vi "TesteTR4CS.vi"() -> ()   [LabVIEW 2024]
uses:
  <vilib>/DAQmx/read.llb/DAQmx Read (Analog DBL 1Chan 1Samp).vi
  <vilib>/DAQmx/miscellaneous.llb/DAQmx Fill In Error Info.vi
panel:
  out "Waveform Chart 3":dbl(graph)
  out "Waveform Chart 2":dbl(graph)
  out "Waveform Chart":dbl(graph)
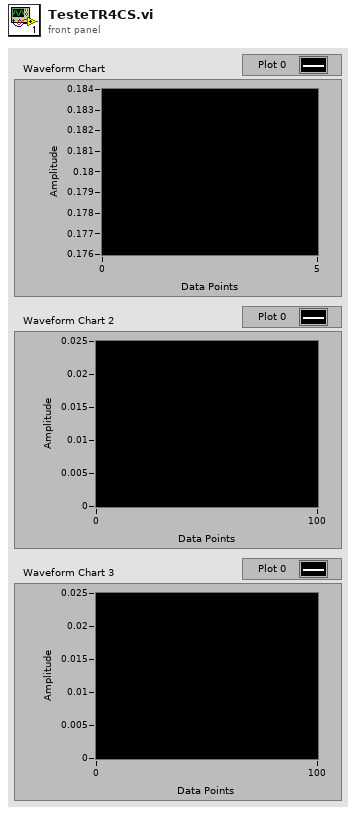
[diagram p1: front panel]
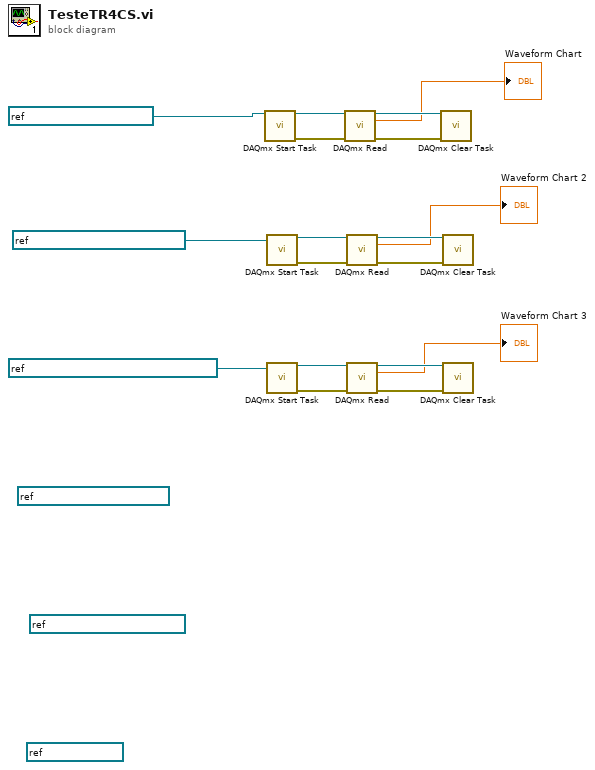
[diagram p0: block diagram]
diagram:
  (unwired) refnum<k21> "CO2_DSO205"
  (unwired) refnum<k21> "Velocidade_Ar_ESV107_1"
  (unwired) refnum<k21> "Termometro_DMA131A"
  n1 = call <vilib>:"DAQmx Start Task.vi"("task/channels in"=refnum<k21> "Luminosidade_ESR000") -> ("task out"=w17:refnum<k21>, "error out"=w15:errorcluster)  [unwired: 13 in]
  n2 = call <vilib>:"DAQmx Start Task.vi"("task/channels in"=refnum<k21> "Radiacao_Solar_PRRDA0130") -> ("task out"=w12:refnum<k21>, "error out"=w9:errorcluster)  [unwired: 13 in]
  n3 = call <vilib>:"DAQmx Start Task.vi"("task/channels in"=refnum<k21> "Temperatura_Umidade_DMA875_1") -> ("task out"=w6:refnum<k21>, "error out"=w3:errorcluster)  [unwired: 13 in]
  n4 = call-poly <vilib>:"DAQmx Read.vi"("task/channels in"=w17, "error in"=w15) -> ("task out"=w16:refnum<k21>, "data"=→"Waveform Chart":dbl, "error out"=w14:errorcluster)  [unwired: 11 in]
  n5 = call-poly <vilib>:"DAQmx Read.vi"("task/channels in"=w12, "error in"=w9) -> ("task out"=w11:refnum<k21>, "data"=→"Waveform Chart 2":dbl, "error out"=w10:errorcluster)  [unwired: 11 in]
  n6 = call-poly <vilib>:"DAQmx Read.vi"("task/channels in"=w6, "error in"=w3) -> ("task out"=w5:refnum<k21>, "data"=→"Waveform Chart 3":dbl, "error out"=w4:errorcluster)  [unwired: 11 in]
  n7 = call <vilib>:"DAQmx Clear Task.vi"("task in"=w16, "error in"=w14) -> ()  [unwired: 13 in, 1 out]
  n8 = call <vilib>:"DAQmx Clear Task.vi"("task in"=w11, "error in"=w10) -> ()  [unwired: 13 in, 1 out]
  n9 = call <vilib>:"DAQmx Clear Task.vi"("task in"=w5, "error in"=w4) -> ()  [unwired: 13 in, 1 out]
